vi "sub_pickup_wf.vi"(10 "b_info":T1, 11 "wf":waveform(dbl) caption="test wf data") -> (3 "pickup_wf":waveform(dbl)(graph) caption="pickup all")   [LabVIEW 2016]
uses:
  <vilib>/Analysis/baseanly.llb/Mean (DBL).vi
  <vilib>/Waveform/WDTOps.llb/WDT Get Waveform Subset DBL.vi
  <vilib>/Waveform/WDTOps.llb/WDT Waveform Duration DBL.vi
  <vilib>/Analysis/baseanly.llb/Unimode.vi
  Global.vi
  <vilib>/measure/mamon.llb/Trigger Detection for 1 Channel.vi
  <vilib>/Analysis/NI_AALBase.lvlib
  <vilib>/measure/NI_MAPro.lvlib
panel:
  in  "탭 컨트롤":enum32{"페이지 1", "페이지 4"}(tab)
  out "standard deviation 2":dbl caption="표준편차" format="%0.2f"
  out "숫자형":i32
  out "chart":cluster{dbl, dbl}(graph)
  out "최빈":cluster{"mode":dbl, dbl, dbl}(graph)
  out "웨이브폼 차트 2":dbl(graph)
  out "detach graph":dbl[](graph)
  out "P_1":waveform(dbl)(graph)
  out "웨이브폼 그래프":dbl[](graph)
  out "next line":bool
  out "zero level":dbl(graph)
  out "pickup back":dbl[](graph)
  out "pickup front":dbl[](graph)
  out "dt":dbl
  out "최빈 max":dbl
  out "mean":dbl caption="평균" format="%0.2f"
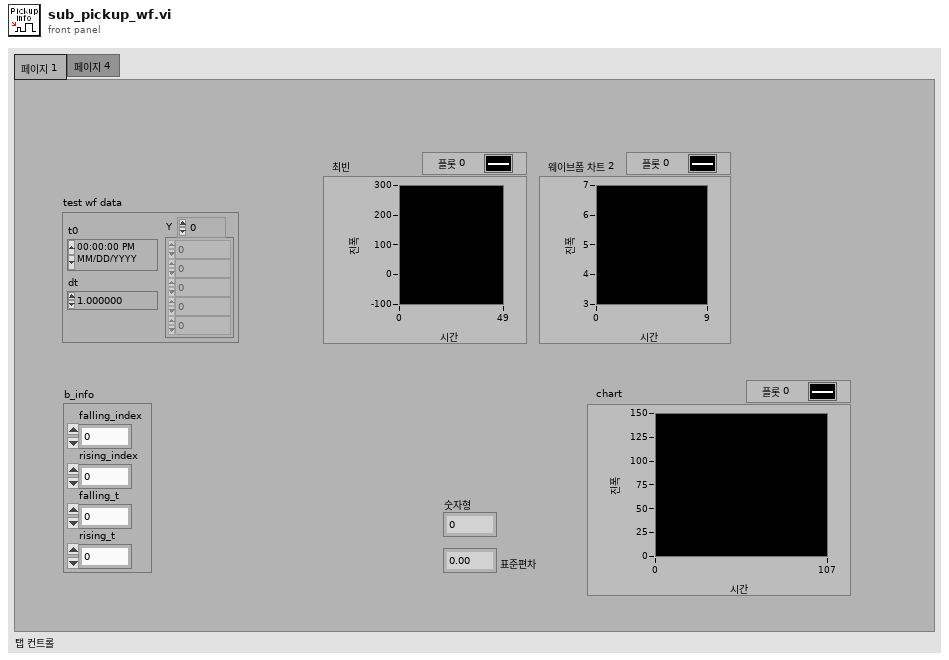
[diagram p1: front panel]
types:
  T1 = cluster{"falling_index":dbl, "rising_index":dbl, "falling_t":dbl, "rising_t":dbl}
  T2 = typedef "data.ctl" = cluster{"Bonding force":dbl, "Bonding time":dbl, "Bonding index":dbl, "Pickup force":dbl, "Pickup time":dbl, "Pickup index":dbl, "Detach force":dbl, "Detach time":dbl, "Detach index":dbl, "Heater temp rt":dbl, "Vacuum rt":dbl, "IR raw data":i16[][], "IR temp data":dbl[][], "vacuum raw wf":waveform(dbl), "vacuum kpa wf":waveform(dbl), "strain raw wf":waveform(dbl)[], "Force rt":dbl, "Vacuum T":dbl, "Heater temp T":dbl, "Balance xy arrays":cluster{dbl, dbl}[], "Balance xy":cluster{dbl, dbl}[], "Bonding wf index":dbl, "Pickup wf index":dbl, "Bonding rising index":dbl, "Bonding falling index":dbl, "Pickup rising index":dbl, "Pickup falling index":dbl}
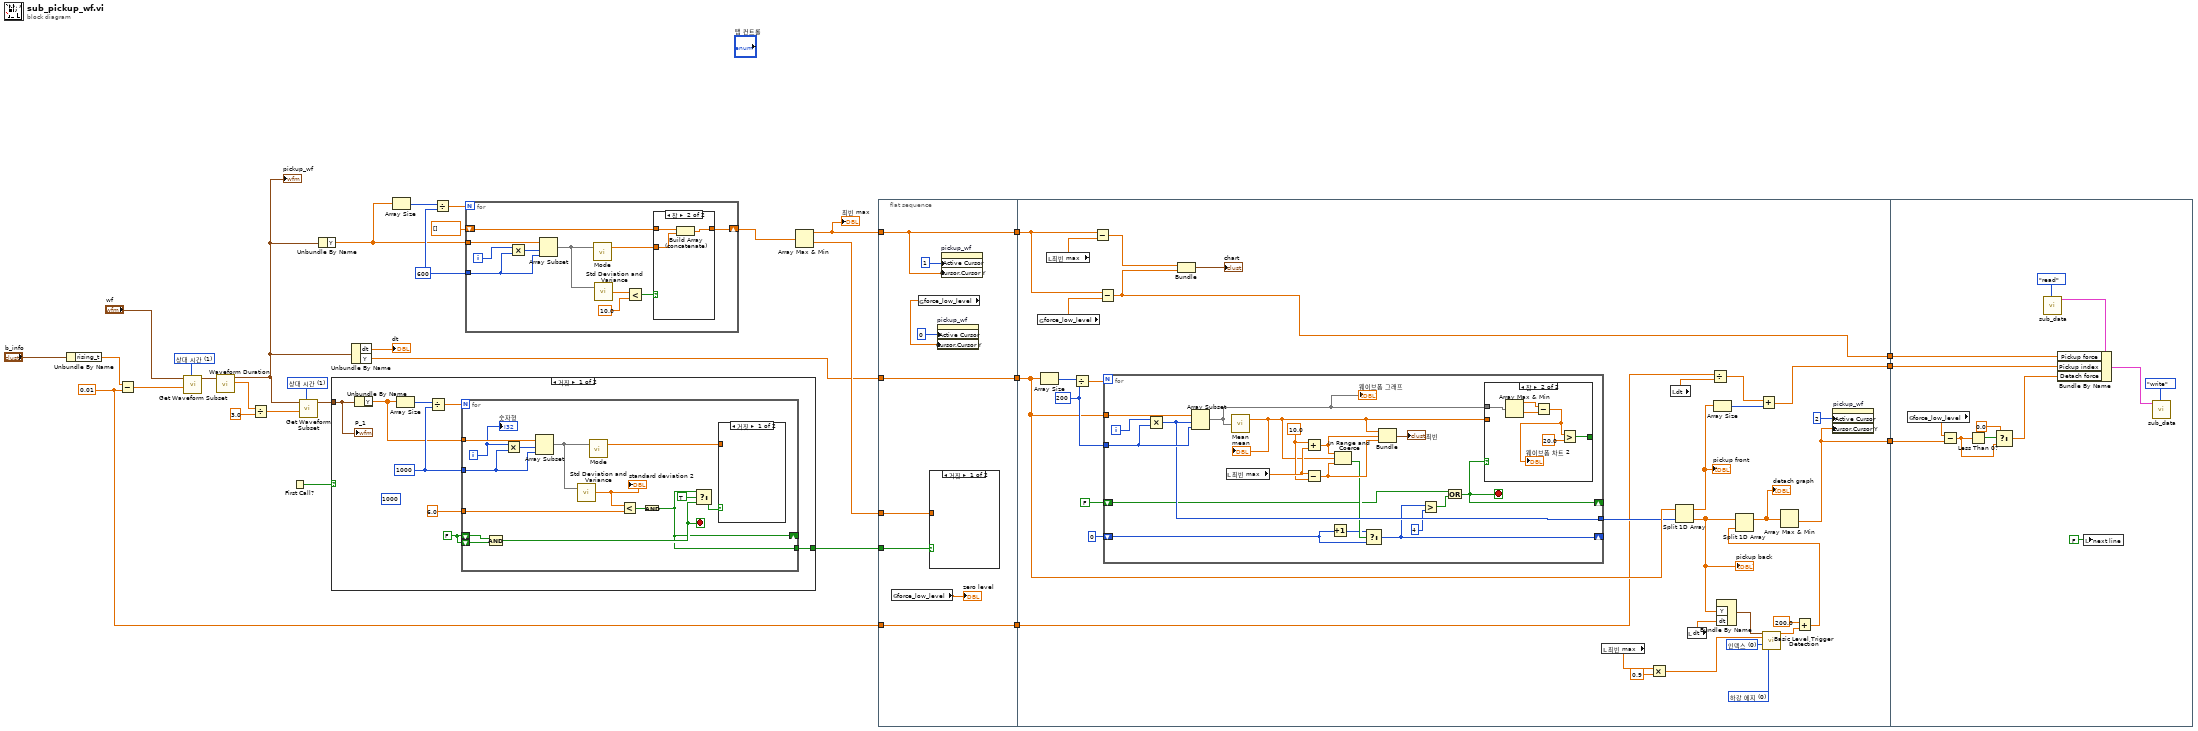
[diagram p0: block diagram]
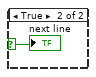
[diagram p2: hidden frame]
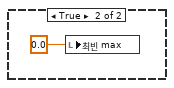
[diagram p3: hidden frame]
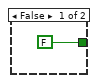
[diagram p6: hidden frame]
diagram:
  w20 = 600 ("block size")
  w23 = u16 1 items=["샘플 ", "상대 시간"] ("start/duration format")
  w2 = 0.01 ("y")
  w24 = u16 1 items=["샘플 ", "상대 시간"] ("start/duration format")
  n1 = Unbundle By Name("b_info") -> ("rising_t"=w26:dbl)
  n2 = Subtract(x=w26, y=w2) -> (x-y=w27:dbl)
  n3 = call-poly <vilib>:"Get Waveform Subset.vi"("start/duration format"=w24, "duration"=w27, "waveform in"="wf") -> ("waveform out"=w25:waveform(dbl))  [unwired: 3 in, 3 out]
  n4 = call-poly <vilib>:"Waveform Duration.vi"("waveform in"=w25) -> ("duration"=w31:dbl, "waveform out"=w9:waveform(dbl))  [unwired: 8 in, 1 out]
  "pickup_wf" <- w9
  n5 = Divide(x=w31, y=3.0) -> (x/y=w22:dbl)
  n6 = First Call?() -> (First Call?: T/F=w5:bool)
  n7 = call-poly <vilib>:"Get Waveform Subset.vi"("start/duration format"=w23, "duration"=w22, "waveform in"=w9) -> ("waveform out"=w21:waveform(dbl))  [unwired: 3 in, 3 out]
  n8 = Unbundle By Name(w9) -> ("Y"=w17:dbl[])
  n9 = case shown="거짓" w5 {
    tunnel: w21 -> [w35 _]
    tunnel: [w34 _] -> w14
    frame False {
      w32 = FALSE
      (unwired) 1000 ("block size")
      w37 = 1000 ("block size")
      n10 = Unbundle By Name(w35) -> ("Y"=w33:dbl[])
      n11 = Array Size(array=w33) -> (size(s)=w38:i32)
      n12 = Divide(x=w38, y=w37) -> (x/y=w39:dbl)
      n13 = for {
        N: w39 -> [_]
        tunnel: w33 -> [w54]
        tunnel: w37 -> [w51]
        tunnel: 6.0 ("y 2") -> [w48]
        tunnel: [w42] -> w34
        shift-right: [w42] -> _
        shift-left: w32 -> [w45]
        shift-left: w32 -> [w44]
        i -> [w52]
        stop <- w43 stop-if-true
        n14 = Compound Arithmetic op=AND(w45, w44) -> (w43:bool)
        n15 = Multiply(x=w52, y=w51) -> (x*y=w53:i32)
        n16 = Array Subset(array=w54, index=w53, length=w51) -> (w50:dbl[])
        n17 = call <vilib>:"Std Deviation and Variance.vi"("X"=w50) -> ("standard deviation"=w49:dbl)  [unwired: 1 in, 2 out]
        "standard deviation 2" <- w49
        n18 = call-poly <vilib>:"Mode.vi"("X"=w50) -> ("mode"=w46:dbl)  [unwired: 1 in, 1 out]
        n19 = Less?(x=w49, y=w48) -> (x < y?=w47:bool)
        n20 = Compound Arithmetic op=AND(w47) -> (w42:bool)
        n21 = Select(t=w42, s=TRUE, f=w43) -> (s? t:f=w41:bool)
        n22 = case shown="거짓" w41 {
          selector: w41 -> [_ w55]
          tunnel: w46 -> [_ _]
          frame False {
          }
          frame True {
            "next line" <- w55
          }
        }
        "숫자형" <- w52
      }
      "P_1" <- w35
    }
    frame True {
      n23 = local write "최빈 max"(0.0 ("최소값")) -> ()
    }
  }
  n24 = Unbundle By Name(w9) -> ("dt"=→"dt":dbl, "Y"=w8:dbl[])
  n25 = Array Size(array=w17) -> (size(s)=w19:i32)
  n26 = Divide(x=w19, y=w20) -> (x/y=w18:dbl)
  n27 = for {
    N: w18 -> [_]
    tunnel: w17 -> [w67]
    tunnel: w20 -> [w64]
    shift-right: [w59] -> w15
    shift-left: dbl[] [] -> [w58]
    i -> [w65]
    n28 = Multiply(x=w65, y=w64) -> (x*y=w66:i32)
    n29 = Array Subset(array=w67, index=w66, length=w64) -> (w63:dbl[])
    n30 = call-poly <vilib>:"Mode.vi"("X"=w63) -> ("mode"=w57:dbl)  [unwired: 1 in, 1 out]
    n31 = call <vilib>:"Std Deviation and Variance.vi"("X"=w63) -> ("standard deviation"=w62:dbl)  [unwired: 1 in, 2 out]
    n32 = Less?(x=w62, y=10.0) -> (x < y?=w60:bool)
    n33 = case shown="참" w60 {
      tunnel: [w68 w71] -> w59
      tunnel: w58 -> [w68 w70]
      tunnel: w57 -> [_ w69]
      frame False {
      }
      frame True {
        n34 = Build Array (concatenate)(w70, w69) -> (w71:dbl[])
      }
    }
  }
  n35 = Array Max & Min(array=w15) -> (max value=w4:dbl, min value=w13:dbl)  [unwired: 2 out]
  "최빈 max" <- w4
  n36 = flat-sequence {
    tunnel: w14 -> [w80]
    tunnel: w13 -> [w79]
    tunnel: w4 -> [w76]
    tunnel: [w76] -> w12
    tunnel: w8 -> [w77]
    tunnel: [w77] -> w11
    tunnel: [w72] -> w3
    tunnel: w2 -> [w72]
    tunnel: w12 -> [w87]
    tunnel: w11 -> [w106]
    tunnel: [w88] -> w10
    tunnel: [w102] -> w7
    tunnel: w3 -> [w83]
    tunnel: [w81] -> w1
    tunnel: w10 -> [w148]
    tunnel: w7 -> [w147]
    tunnel: w1 -> [w140]
    frame #0 {
      n37 = global read "Global.vi" "force_low_level"() -> (→"zero level":dbl)
      n38 = global read "Global.vi" "force_low_level"() -> (w74:dbl)
      n39 = case shown="거짓" w80 {
        tunnel: w79 -> [_ _]
        frame False {
        }
        frame True {
        }
      }
      n40 = property on="pickup_wf" class="WFGraph (엄격한)"("Active Cursor"=u32 0 ("활성 커서"), "Cursor.Cursor Y"=w74) -> ()  [unwired: 2 in, 2 out]
      n41 = property on="pickup_wf" class="WFGraph (엄격한)"("Active Cursor"=u32 1 ("활성 커서"), "Cursor.Cursor Y"=w76) -> ()  [unwired: 2 in, 2 out]
    }
    frame #1 {
      w94 = u16 0 items=["하강 에지", "상승 에지"] ("trigger slope")
      w95 = u16 0 items=["인덱스", "시간"] ("location mode")
      w108 = 200 ("block size")
      n42 = global read "Global.vi" "force_low_level"() -> (w112:dbl)
      n43 = Array Size(array=w106) -> (size(s)=w110:i32)
      n44 = local read "최빈 max"() -> (w113:dbl)
      n45 = Divide(x=w110, y=w108) -> (x/y=w109:dbl)
      n46 = Subtract(x=w87, y=w113) -> (x-y=w90:dbl)
      n47 = Subtract(x=w87, y=w112) -> (x-y=w88:dbl)
      n48 = for {
        N: w109 -> [_]
        tunnel: w106 -> [w132]
        tunnel: w108 -> [w130]
        shift-right: [w114] -> _
        shift-left: FALSE -> [w118]
        tunnel: [w126] -> w105
        shift-right: [w117] -> _
        shift-left: 0 ("block size") -> [w119]
        i -> [w131]
        stop <- w114 stop-if-true
        w127 = 10.0 ("x")
        n49 = Multiply(x=w131, y=w130) -> (x*y=w126:i32)
        n50 = Array Subset(array=w132, index=w126, length=w130) -> (w129:dbl[])
        "웨이브폼 그래프" <- w129
        n51 = local read "최빈 max"() -> (w128:dbl)
        n52 = call-poly <vilib>:"Mean.vi"("X"=w129) -> ("mean"=w125:dbl)  [unwired: 1 out]
        "mean" <- w125
        n53 = Add(x=w127, y=w128) -> (x+y=w124:dbl)
        n54 = Subtract(x=w128, y=w127) -> (x-y=w123:dbl)
        n55 = Increment(x=w119) -> (x+1=w120:i32)
        n56 = In Range and Coerce(upper limit=w124, x=w125, lower limit=w123) -> (In Range?=w121:bool)  [unwired: 1 out]
        n57 = Select(t=w120, s=w121, f=w119) -> (s? t:f=w117:i32)
        n58 = Bundle("mean"=w125, w124, w123) -> (→"최빈":cluster{"mean":dbl, dbl, dbl})  [unwired: 1 in]
        n59 = Greater?(x=w117, y=4) -> (0:w115:bool)
        n60 = Or(x=w118, y=w115) -> (x .or. y?=w114:bool)
        n61 = case shown="참" w114 {
          tunnel: w125 -> [_ _]
          tunnel: w129 -> [_ w137]
          tunnel: [FALSE w138] -> _
          frame False {
          }
          frame True {
            n62 = Array Max & Min(array=w137) -> (max value=w136:dbl, min value=w135:dbl)  [unwired: 2 out]
            n63 = Subtract(x=w136, y=w135) -> (x-y=w134:dbl)
            "웨이브폼 차트 2" <- w134
            n64 = Greater?(x=w134, y=20.0) -> (0:w138:bool)
          }
        }
      }
      n65 = Bundle(w90, w88) -> (→"chart":cluster{dbl, dbl})  [unwired: 1 in]
      n66 = local read "최빈 max"() -> (w98:dbl)
      n67 = Multiply(x=w98, y=0.9) -> (x*y=w96:dbl)
      n68 = local read "dt"() -> (w84:dbl)
      n69 = Split 1D Array(array=w106, index=w105) -> (first subarray=w86:dbl[], second subarray=w101:dbl[])
      "pickup front" <- w86
      "pickup back" <- w101
      n70 = local read "dt"() -> (w100:dbl)
      n71 = Divide(x=w83, y=w84) -> (x/y=w82:dbl)
      n72 = Array Size(array=w86) -> (size(s)=w85:i32)
      n73 = Bundle By Name("Y"=w101, "dt"=w100) -> (w99:waveform(dbl))  [unwired: 1 in]
      n74 = Add(x=w82, y=w85) -> (x+y=w81:dbl)
      n75 = call-poly <vilib>:"Basic Level Trigger Detection.vi"("signal in"=w99, "level"=w96, "location mode"=w95, "trigger slope"=w94) -> ("trigger location"=w93:dbl)  [unwired: 9 in, 2 out]
      n76 = Add(x=200.0, y=w93) -> (x+y=w91:dbl)
      n77 = Split 1D Array(array=w101, index=w91) -> (first subarray=w89:dbl[])  [unwired: 1 out]
      "detach graph" <- w89
      n78 = Array Max & Min(array=w89) -> (min value=w102:dbl)  [unwired: 3 out]
      n79 = property on="pickup_wf" class="WFGraph (엄격한)"("Active Cursor"=u32 2 ("활성 커서"), "Cursor.Cursor Y"=w102) -> ()  [unwired: 2 in, 2 out]
    }
    frame #2 {
      n80 = global read "Global.vi" "force_low_level"() -> (w146:dbl)
      n81 = Subtract(x=w146, y=w147) -> (x-y=w144:dbl)
      n82 = Less Than 0?(x=w144) -> (x < 0?=w145:bool)
      n83 = Select(t=0.0, s=w145, f=w144) -> (s? t:f=w142:dbl)
      n84 = call "sub_data.vi"("cmd"=enum16{"ini", "write", "read"}."read") -> ("data out"=w150:T2)  [unwired: 9 in, 1 out]
      n85 = Bundle By Name(cluster=w150, "Pickup force"=w148, "Pickup index"=w140, "Detach force"=w142) -> (w152:T2)
      n86 = local write "next line"(FALSE ("next line")) -> ()
      n87 = call "sub_data.vi"("cmd"=enum16{"ini", "write", "read"}."write", "data in"=w152) -> ()  [unwired: 8 in, 2 out]
    }
  }
